vi "input_alive.vi"(8 "error in (no error)":errorcluster, 11 "input_poller in":refnum<class "input_poller.lvclass">) -> (0 "error out":errorcluster, 2 "alive":bool, 3 "input_poller out":refnum<class "input_poller.lvclass">)   [LabVIEW 2015, in "input_poller.lvclass"]
uses:
  input_poller.lvclass
  input_poller.lvclass/input_poller.ctl
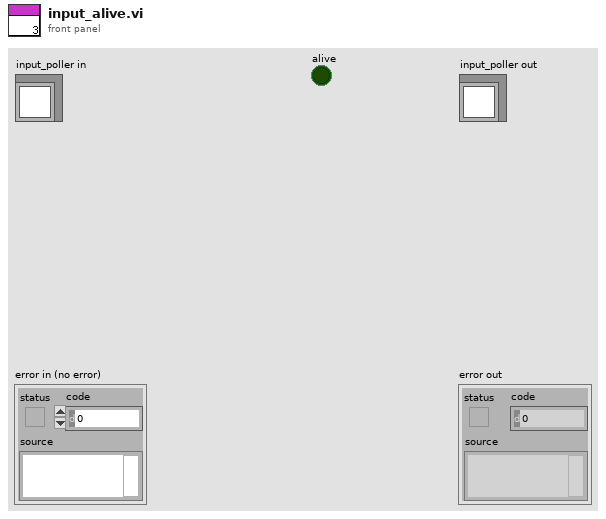
[diagram p1: front panel]
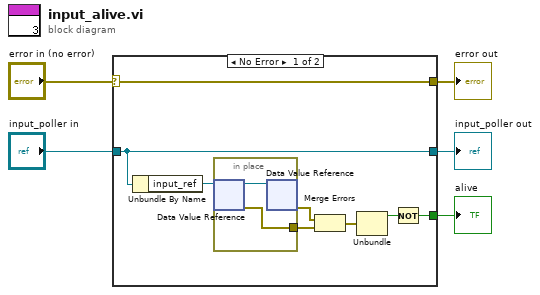
[diagram p0: block diagram]
diagram:
  n1 = case shown="No Error" "error in (no error)" {
    selector: "error in (no error)" -> [w13 w17]
    tunnel: [w13 w17] -> w4
    tunnel: [w7 w16] -> w2
    tunnel: "input_poller in" -> [w7 w16]
    tunnel: [w6 _] -> w1
    frame No Error {
      n2 = Unbundle By Name(w7) -> ("input_ref"=w12:refnum<data-value>)
      n3 = in-place {
        in-place-border: [w14] -> w10
        n4 = in-place-dvr #1(w12) -> (w15:refnum<class "input.lvclass">, w14:errorcluster)
        n5 = in-place-dvr #1(w15) -> (w11:errorcluster)  [unwired: 1 out]
      }
      n6 = Merge Errors(w11, w10) -> (w9:errorcluster)
      n7 = Unbundle(w9) -> ("status"=w8:bool)  [unwired: 2 out]
      n8 = Not(x=w8) -> (.not. x?=w6:bool)
    }
    frame Error {
    }
  }
  "error out" <- w4
  "input_poller out" <- w2
  "alive" <- w1
